vi "Drive Core.vi"(0 "A Encoder BL":string="My Motor RefNum", 1 "Rotational Motor FR":string="My Motor RefNum", 2 "Rotational Motor FL":string="My Motor RefNum", 3 "Rotational Motor BR":string="My Motor RefNum", 4 "Rotational Motor BL":string="My Motor RefNum", 5 "Drive Motor FR":string="My Motor RefNum", 6 "A Encoder BR":string="My Motor RefNum", 7 "Drive Motor FL":string="My Motor RefNum", 8 "A Encoder FL":string="My Motor RefNum", 9 "Drive Motor BR":string="My Motor RefNum", 10 "A Encoder FR":string="My Motor RefNum", 11 "Drive Motor BL":string="My Motor RefNum") -> ()   [LabVIEW 2014]
uses:
  Global Variables.vi
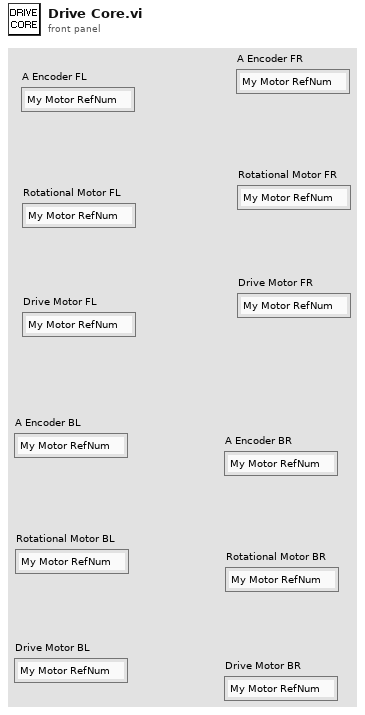
[diagram p1: front panel]
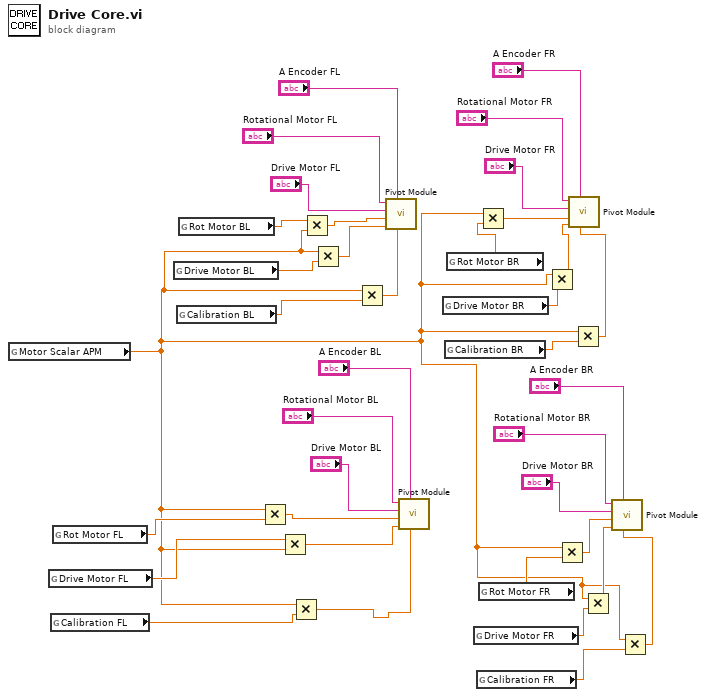
[diagram p0: block diagram]
diagram:
  n1 = global read "Global Variables.vi" "Motor Scalar APM"() -> (w2:dbl)
  n2 = global read "Global Variables.vi" "Drive Motor FL"() -> (w17:dbl)
  n3 = global read "Global Variables.vi" "Calibration FL"() -> (w19:dbl)
  n4 = global read "Global Variables.vi" "Rot Motor FL"() -> (w14:dbl)
  n5 = global read "Global Variables.vi" "Drive Motor BL"() -> (w23:dbl)
  n6 = global read "Global Variables.vi" "Calibration BL"() -> (w25:dbl)
  n7 = global read "Global Variables.vi" "Rot Motor BL"() -> (w21:dbl)
  n8 = Multiply(x=w2, y=w14) -> (x*y=w15:dbl)
  n9 = Multiply(x=w17, y=w2) -> (x*y=w16:dbl)
  n10 = Multiply(x=w2, y=w19) -> (x*y=w18:dbl)
  n11 = Multiply(x=w21, y=w2) -> (x*y=w20:dbl)
  n12 = Multiply(x=w2, y=w23) -> (x*y=w22:dbl)
  n13 = Multiply(x=w2, y=w25) -> (x*y=w24:dbl)
  n14 = call "Pivot Module.vi"("Calibration Angle"=w24, "Encoder Refnum"="A Encoder FL", "Motor Speed"=w22, "Motor Angle"=w20, "Drive Motor Refnum"="Drive Motor FL", "Rotational Motor Refnum"="Rotational Motor FL") -> ()  [unwired: 6 in]
  n15 = call "Pivot Module.vi"("Calibration Angle"=w18, "Encoder Refnum"="A Encoder BL", "Motor Speed"=w16, "Motor Angle"=w15, "Drive Motor Refnum"="Drive Motor BL", "Rotational Motor Refnum"="Rotational Motor BL") -> ()  [unwired: 6 in]
  n16 = global read "Global Variables.vi" "Drive Motor BR"() -> (w11:dbl)
  n17 = global read "Global Variables.vi" "Calibration BR"() -> (w9:dbl)
  n18 = global read "Global Variables.vi" "Rot Motor BR"() -> (w13:dbl)
  n19 = global read "Global Variables.vi" "Drive Motor FR"() -> (w5:dbl)
  n20 = global read "Global Variables.vi" "Calibration FR"() -> (w3:dbl)
  n21 = Multiply(x=w2, y=w13) -> (x*y=w12:dbl)
  n22 = global read "Global Variables.vi" "Rot Motor FR"() -> (w7:dbl)
  n23 = Multiply(x=w2, y=w11) -> (x*y=w10:dbl)
  n24 = Multiply(x=w2, y=w7) -> (x*y=w6:dbl)
  n25 = Multiply(x=w2, y=w9) -> (x*y=w8:dbl)
  n26 = call "Pivot Module.vi"("Calibration Angle"=w8, "Encoder Refnum"="A Encoder FR", "Motor Speed"=w10, "Motor Angle"=w12, "Drive Motor Refnum"="Drive Motor FR", "Rotational Motor Refnum"="Rotational Motor FR") -> ()  [unwired: 6 in]
  n27 = Multiply(x=w2, y=w5) -> (x*y=w4:dbl)
  n28 = Multiply(x=w2, y=w3) -> (x*y=w1:dbl)
  n29 = call "Pivot Module.vi"("Calibration Angle"=w1, "Encoder Refnum"="A Encoder BR", "Motor Speed"=w4, "Motor Angle"=w6, "Drive Motor Refnum"="Drive Motor BR", "Rotational Motor Refnum"="Rotational Motor BR") -> ()  [unwired: 6 in]
